vi "ReadFilterINI (SubVI).vi"(9 "CheckMD5":bool, 10 "base path":path, 11 "md5":string) -> (0 "HPF1":cluster{"Frq":dbl[], "Kt":dbl[]}[](array[cluster]), 1 "LPF1":cluster{"Frq":dbl[], "Kt":dbl[]}[](array[cluster]), 2 "HPF0":cluster{"Frq":dbl[], "Kt":dbl[]}[](array[cluster]), 3 "LPF0":cluster{"Frq":dbl[], "Kt":dbl[]}[](array[cluster]))   [LabVIEW 2017]
uses:
  <vilib>/Utility/config.llb/NI_LVConfig.lvlib
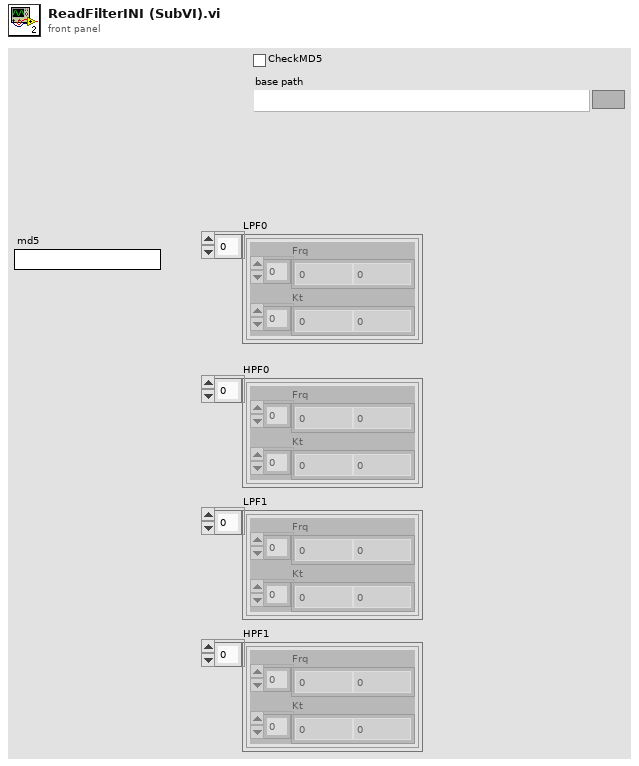
[diagram p1: front panel]
types:
  T1 = typedef "NI_LVConfig.lvlib/Config Data RefNum.ctl" = refnum<k1>
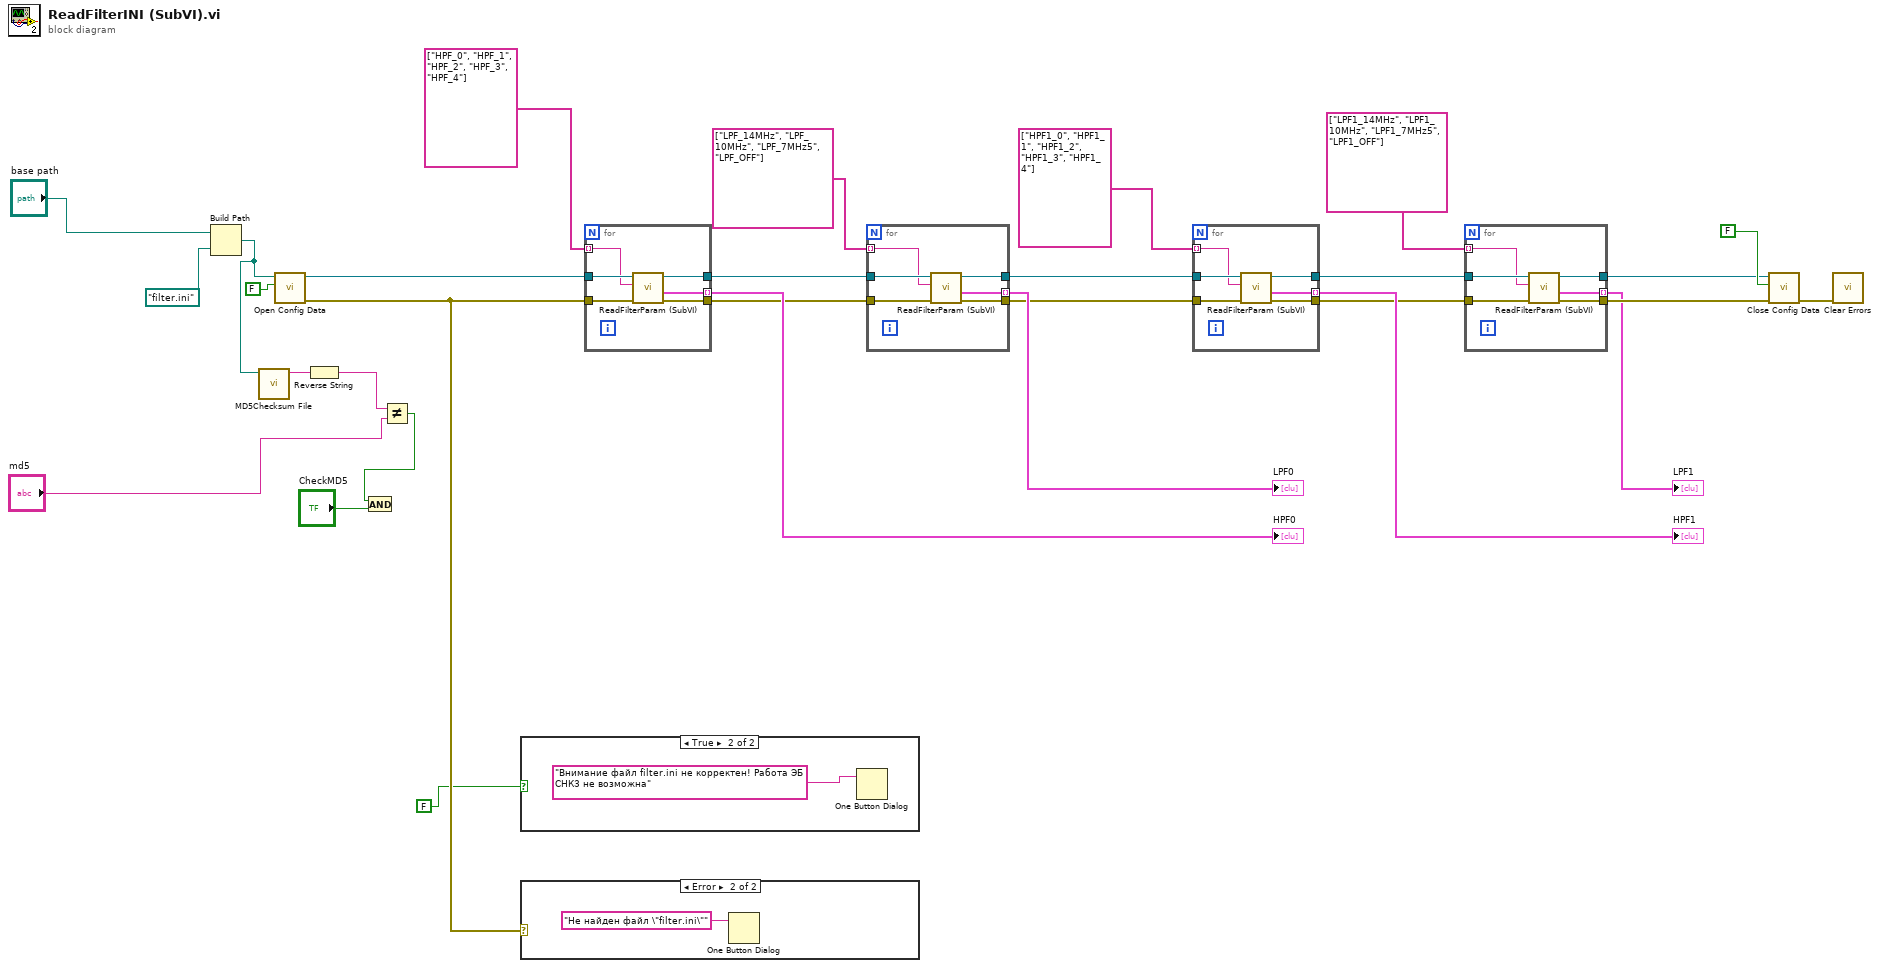
[diagram p0: block diagram]
diagram:
  n1 = Build Path(base path="base path", name or relative path=path "filter.ini" ("default name")) -> (appended path=w26:path)
  n2 = call <vilib>:"MD5Checksum File.vi"("Path"=w26) -> ("MD5 message-digest"=w27:string)  [unwired: 9 in, 1 out]
  n3 = call <vilib>:"Open Config Data.vi"("create file if necessary (T)"=FALSE ("create file if necessary? (T)"), "configuration file path"=w26) -> ("error out"=w30:errorcluster, "refnum"=w22:T1)  [unwired: 7 in, 1 out]
  n4 = Reverse String(1:w27) -> (0:w28:string)
  n5 = Not Equal?(x=w28, y="md5") -> (x != y?=w13:bool)
  n6 = And(x=w13, y="CheckMD5") -> ()  [unwired: 1 out]
  n7 = case shown="True" FALSE {
    frame False {
    }
    frame True {
      n8 = One Button Dialog(message="Внимание файл filter.ini не корректен! Работа ЭБ СНК3 не возможна") -> ()  [unwired: 1 in, 1 out]
    }
  }
  n9 = case shown="Error" w30 {
    frame No Error {
    }
    frame Error {
      n10 = One Button Dialog(message="Не найден файл \"filter.ini\"") -> ()  [unwired: 1 in, 1 out]
    }
  }
  n11 = for {
    tunnel: string[] ["HPF_0", "HPF_1", "HPF_2", "HPF_3", "HPF_4"] ("Array 2") -> [w34] mode=indexing
    tunnel: w22 -> [w38]
    tunnel: [w36] -> w18
    tunnel: w30 -> [w37]
    tunnel: [w35] -> w19
    tunnel: [w33] -> w21 mode=indexing
    n12 = call "ReadFilterParam (SubVI).vi"("error in (no error)"=w37, "section"=w34, "Refnum in"=w38) -> ("error out"=w35:errorcluster, "BodePlot"=w33:cluster{"Frq":dbl[], "Kt":dbl[]}, "Refnum out"=w36:T1)  [unwired: 6 in]
  }
  "HPF0" <- w21
  n13 = for {
    tunnel: string[] ["LPF_14MHz", "LPF_10MHz", "LPF_7MHz5", "LPF_OFF"] ("Array") -> [w40] mode=indexing
    tunnel: w18 -> [w44]
    tunnel: [w42] -> w10
    tunnel: w19 -> [w43]
    tunnel: [w41] -> w9
    tunnel: [w39] -> w17 mode=indexing
    n14 = call "ReadFilterParam (SubVI).vi"("error in (no error)"=w43, "section"=w40, "Refnum in"=w44) -> ("error out"=w41:errorcluster, "BodePlot"=w39:cluster{"Frq":dbl[], "Kt":dbl[]}, "Refnum out"=w42:T1)  [unwired: 6 in]
  }
  "LPF0" <- w17
  n15 = for {
    tunnel: string[] ["HPF1_0", "HPF1_1", "HPF1_2", "HPF1_3", "HPF1_4"] ("Array 2") -> [w46] mode=indexing
    tunnel: w10 -> [w50]
    tunnel: [w48] -> w6
    tunnel: w9 -> [w49]
    tunnel: [w47] -> w7
    tunnel: [w45] -> w8 mode=indexing
    n16 = call "ReadFilterParam (SubVI).vi"("error in (no error)"=w49, "section"=w46, "Refnum in"=w50) -> ("error out"=w47:errorcluster, "BodePlot"=w45:cluster{"Frq":dbl[], "Kt":dbl[]}, "Refnum out"=w48:T1)  [unwired: 6 in]
  }
  "HPF1" <- w8
  n17 = for {
    tunnel: string[] ["LPF1_14MHz", "LPF1_10MHz", "LPF1_7MHz5", "LPF1_OFF"] ("Array") -> [w52] mode=indexing
    tunnel: w6 -> [w56]
    tunnel: [w54] -> w5
    tunnel: w7 -> [w55]
    tunnel: [w53] -> w4
    tunnel: [w51] -> w2 mode=indexing
    n18 = call "ReadFilterParam (SubVI).vi"("error in (no error)"=w55, "section"=w52, "Refnum in"=w56) -> ("error out"=w53:errorcluster, "BodePlot"=w51:cluster{"Frq":dbl[], "Kt":dbl[]}, "Refnum out"=w54:T1)  [unwired: 6 in]
  }
  "LPF1" <- w2
  n19 = call <vilib>:"Close Config Data.vi"("error in (no error)"=w4, "write file if changed (T)"=FALSE ("write configuration file? (T)"), "refnum"=w5) -> ("error out"=w24:errorcluster)  [unwired: 8 out]
  n20 = call <vilib>:"Clear Errors.vi"("error in (no error)"=w24) -> ()  [unwired: 5 in, 2 out]
